vi "Client2.vi"() -> ()   [LabVIEW 2016]
uses:
  <vilib>/Utility/tcp.llb/UDP Multicast Read-Only Open.vi
panel:
  out "MA_Validation":u8
  out "IsNotConnected?":bool
  in  "LeaveServer":bool
  out "Greetings":string
  in  "Exit":bool
  out "MulticastAddress":string
  out "AuthKey":string
  in  "Connect":bool
  in  "Server Port":u32
  in  "Server IP":string
  in  "Send":bool
  in  "Chat_Insert":string
  out "Chat":string
  # "Server IP-Adress"
  # "Server Port"
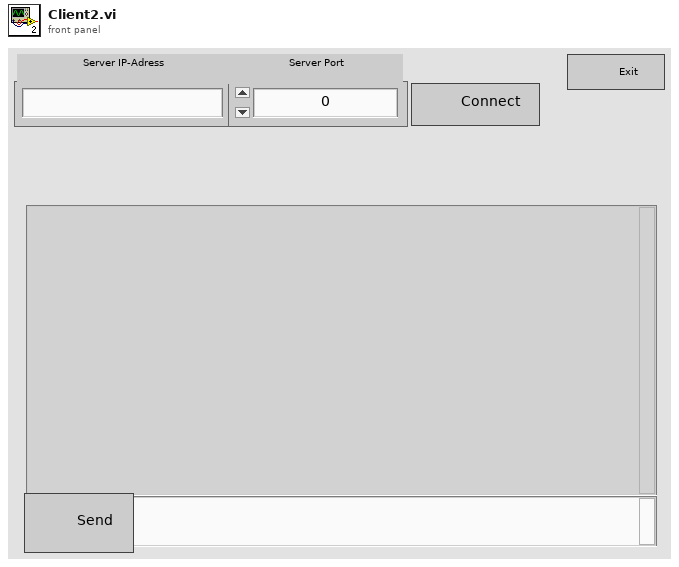
[diagram p1: front panel]
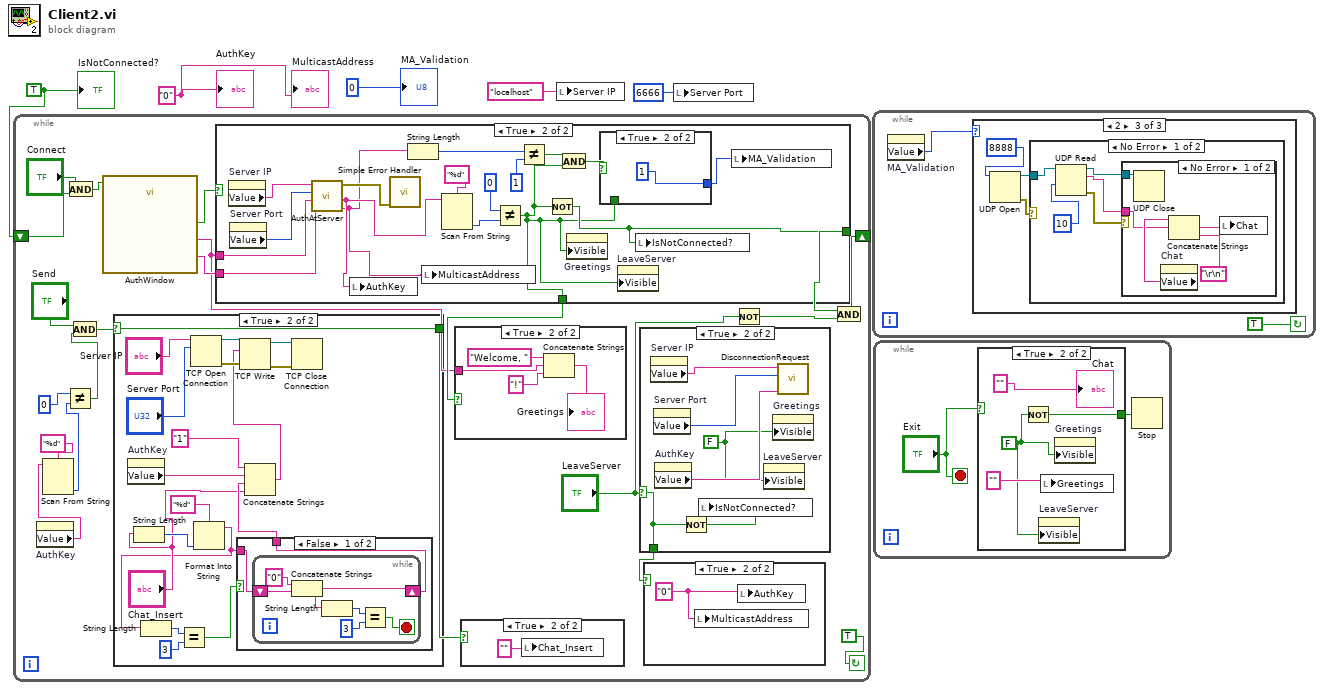
[diagram p0: block diagram]
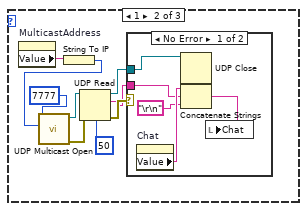
[diagram p3: hidden frame]
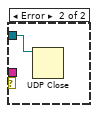
[diagram p5: hidden frame]
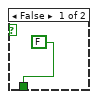
[diagram p9: hidden frame]
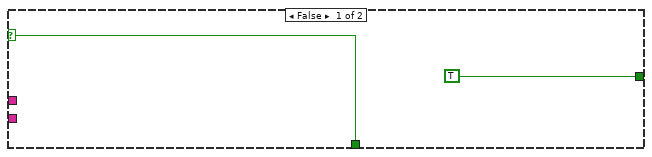
[diagram p14: hidden frame]
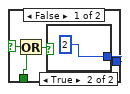
[diagram p15: hidden frame]
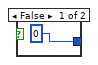
[diagram p16: hidden frame]
diagram:
  w1 = TRUE
  w2 = "0"
  n1 = while {
    shift-right: [w9] -> _
    shift-left: w1 -> [w8]
    stop <- TRUE continue-if-true
    n2 = property on="AuthKey" class="Str"() -> ("Value"=w20:string)  [unwired: 2 in, 2 out]
    n3 = Scan From String(format string="%d", input string=w20) -> (output 1=w18:i32)  [unwired: 3 in, 3 out]
    n4 = Not Equal?(x=0, y=w18) -> (x != y?=w15:bool)
    n5 = And(x="Connect", y=w8) -> (x .and. y?=w13:bool)
    n6 = And(x="Send", y=w15) -> (x .and. y?=w16:bool)
    n7 = call "AuthWindow.vi"("Enable"=w13) -> ("Password"=w23:string, "Login"=w22:string, "Enter"=w21:bool)  [unwired: 15 in, 1 out]
    n8 = case shown="True" w16 {
      selector: w16 -> [w40 w54]
      tunnel: [w40 w54] -> w25
      frame False {
      }
      frame True {
        n9 = property on="AuthKey" class="Str"() -> ("Value"=w45:string)  [unwired: 2 in, 2 out]
        n10 = String Length(string="Chat_Insert") -> (length=w56:i32)
        n11 = TCP Open Connection(address="Server IP", remote port or service name="Server Port") -> (connection ID=w46:refnum<k5>, error out=w47:errorcluster)  [unwired: 3 in]
        n12 = Format Into String(format string="%d", w56) -> (resulting string=w48:string)  [unwired: 2 in, 1 out]
        n13 = String Length(string=w48) -> (length=w52:i32)
        n14 = Equal?(x=w52, y=3) -> (x = y?=w51:bool)
        n15 = case shown="False" w51 {
          tunnel: w48 -> [w60 w67]
          tunnel: [w59 w67] -> w50
          frame False {
            n16 = while {
              shift-right: [w62] -> w59
              shift-left: w60 -> [w66]
              stop <- w61 stop-if-true
              n17 = Concatenate Strings("0", w66) -> (w62:string)
              n18 = String Length(string=w62) -> (length=w63:i32)
              n19 = Equal?(x=w63, y=3) -> (x = y?=w61:bool)
            }
          }
          frame True {
          }
        }
        n20 = Concatenate Strings("1", w45, w50, "Chat_Insert") -> (w43:string)
        n21 = TCP Write(connection ID=w46, data in=w43, error in (no error)=w47) -> (connection ID out=w42:refnum<k5>, error out=w41:errorcluster)  [unwired: 1 in, 1 out]
        n22 = TCP Close Connection(connection ID=w42, error in (no error)=w41) -> ()  [unwired: 1 in, 2 out]
      }
    }
    n23 = case shown="True" w21 {
      selector: w21 -> [w69 _]
      tunnel: w22 -> [_ w83]
      tunnel: w23 -> [_ w82]
      tunnel: [w69 w72] -> w24
      tunnel: [TRUE w77] -> w6
      frame False {
      }
      frame True {
        n24 = property on="Server IP" class="Str"() -> ("Value"=w85:string)  [unwired: 2 in, 2 out]
        n25 = property on="Server Port" class="DigNum (strict)"() -> ("Value"=w84:u32)  [unwired: 2 in, 2 out]
        n26 = call "AuthAtServer.vi"("password"=w82, "login"=w83, "Port"=w84, "Adress"=w85) -> ("MulticastAdress"=w75:string, "AuthKey"=w78:string, "error out"=w86:errorcluster)  [unwired: 5 in]
        n27 = local write "AuthKey"(w78) -> ()
        n28 = call <vilib>:"Simple Error Handler.vi"("error in (no error)"=w86) -> ()  [unwired: 4 in, 5 out]
        n29 = String Length(string=w75) -> (length=w74:i32)
        n30 = local write "MulticastAddress"(w75) -> ()
        n31 = Scan From String(format string="%d", input string=w78) -> (output 1=w80:i32)  [unwired: 3 in, 3 out]
        n32 = Not Equal?(x=0, y=w80) -> (x != y?=w72:bool)
        n33 = Not Equal?(x=w74, y=1) -> (x != y?=w71:bool)
        n34 = Not(x=w72) -> (.not. x?=w77:bool)
        n35 = And(x=w71, y=w72) -> (x .and. y?=w73:bool)
        n36 = property on="Greetings" class="Str"("Visible"=w72) -> ()  [unwired: 2 in, 2 out]
        n37 = case shown="True" w73 {
          selector: w73 -> [w87 _]
          tunnel: [w90 1] -> w70
          tunnel: w72 -> [w89 _]
          frame False {
            n38 = Or(x=w87, y=w89) -> (x .or. y?=w88:bool)
            n39 = case shown="True" w88 {
              tunnel: [0 2] -> w90
              frame False {
              }
              frame True {
              }
            }
          }
          frame True {
          }
        }
        n40 = property on="LeaveServer" class="Bool"("Visible"=w72) -> ()  [unwired: 2 in, 2 out]
        n41 = local write "IsNotConnected?"(w77) -> ()
        n42 = local write "MA_Validation"(w70) -> ()
      }
    }
    n43 = case shown="True" w24 {
      tunnel: w22 -> [_ w37]
      frame False {
      }
      frame True {
        n44 = Concatenate Strings("Welcome, ", w37, "!") -> (→"Greetings":string)
      }
    }
    n45 = case shown="True" w25 {
      frame False {
      }
      frame True {
        n46 = local write "Chat_Insert"("") -> ()
      }
    }
    n47 = case shown="True" "LeaveServer" {
      selector: "LeaveServer" -> [_ w31]
      tunnel: [FALSE w31] -> w11
      frame False {
      }
      frame True {
        w29 = FALSE
        n48 = property on="Server IP" class="Str"() -> ("Value"=w34:string)  [unwired: 2 in, 2 out]
        n49 = property on="Server Port" class="DigNum (strict)"() -> ("Value"=w33:u32)  [unwired: 2 in, 2 out]
        n50 = property on="AuthKey" class="Str"() -> ("Value"=w32:string)  [unwired: 2 in, 2 out]
        n51 = Not(x=w31) -> (.not. x?=w30:bool)
        n52 = local write "IsNotConnected?"(w30) -> ()
        n53 = property on="LeaveServer" class="Bool"("Visible"=w29) -> ()  [unwired: 2 in, 2 out]
        n54 = property on="Greetings" class="Str"("Visible"=w29) -> ()  [unwired: 2 in, 2 out]
        n55 = call "DisconnectionRequest.vi"("AuthKey"=w32, "Server Port"=w33, "Server IP"=w34) -> ()  [unwired: 9 in]
      }
    }
    n56 = case shown="True" w11 {
      frame False {
      }
      frame True {
        w27 = "0"
        n57 = local write "MulticastAddress"(w27) -> ()
        n58 = local write "AuthKey"(w27) -> ()
      }
    }
    n59 = Not(x="LeaveServer") -> (.not. x?=w7:bool)
    n60 = And(x=w6, y=w7) -> (x .and. y?=w9:bool)
  }
  n61 = local write "Server IP"("localhost") -> ()
  n62 = local write "Server Port"(u16 6666) -> ()
  n63 = while {
    stop <- TRUE continue-if-true
    n64 = property on="MA_Validation" class="DigNum (strict)"() -> ("Value"=w94:u8)  [unwired: 2 in, 2 out]
    n65 = case shown="2" w94 {
      frame 0, Default {
      }
      frame 1 {
        n66 = property on="MulticastAddress" class="Str"() -> ("Value"=w103:string)  [unwired: 2 in, 2 out]
        n67 = String To IP(1:w103) -> (0:w102:u32)
        n68 = call-poly <vilib>:"UDP Multicast Open.vi"("multicast addr"=w102, "port"=7777) -> ("error out"=w100:errorcluster, "connection ID"=w101:refnum<k16>)  [unwired: 7 in, 1 out]
        n69 = UDP Read(connection ID=w101, timeout ms (25000)=50, 8:w100) -> (data out=w96:string, error out=w97:errorcluster, 3:w98:refnum<k16>)  [unwired: 1 in, 2 out]
        n70 = case shown="No Error" w97 {
          tunnel: w98 -> [w106 _]
          tunnel: w96 -> [w105 _]
          frame No Error {
            n71 = property on="Chat" class="Str"() -> ("Value"=w109:string)  [unwired: 2 in, 2 out]
            n72 = UDP Close(connection ID=w106) -> ()  [unwired: 1 in, 2 out]
            n73 = Concatenate Strings(w109, w105, "\r\n") -> (w108:string)
            n74 = local write "Chat"(w108) -> ()
          }
          frame Error {
          }
        }
      }
      frame 2 {
        n75 = UDP Open(11:8888) -> (port=w111:refnum<k16>, 0:w112:errorcluster)  [unwired: 4 in, 1 out]
        n76 = case shown="No Error" w112 {
          tunnel: w111 -> [w117 _]
          frame No Error {
            n77 = UDP Read(connection ID=w117, timeout ms (25000)=10) -> (data out=w114:string, error out=w115:errorcluster, 3:w116:refnum<k16>)  [unwired: 2 in, 2 out]
            n78 = case shown="No Error" w115 {
              tunnel: w116 -> [w119 w123]
              tunnel: w114 -> [w118 _]
              frame No Error {
                n79 = UDP Close(connection ID=w119) -> ()  [unwired: 1 in, 2 out]
                n80 = property on="Chat" class="Str"() -> ("Value"=w122:string)  [unwired: 2 in, 2 out]
                n81 = Concatenate Strings(w122, w118, "\r\n") -> (w120:string)
                n82 = local write "Chat"(w120) -> ()
              }
              frame Error {
                n83 = UDP Close(connection ID=w123) -> ()  [unwired: 1 in, 2 out]
              }
            }
          }
          frame Error {
          }
        }
      }
    }
  }
  n84 = while {
    stop <- "Exit" stop-if-true
    n85 = case shown="True" "Exit" {
      selector: "Exit" -> [w126 _]
      tunnel: [w126 w129] -> w124
      frame False {
      }
      frame True {
        w128 = FALSE
        n86 = Not(x=w128) -> (.not. x?=w129:bool)
        n87 = property on="LeaveServer" class="Bool"("Visible"=w128) -> ()  [unwired: 2 in, 2 out]
        n88 = local write "Greetings"("") -> ()
        n89 = property on="Greetings" class="Str"("Visible"=w128) -> ()  [unwired: 2 in, 2 out]
        "Chat" <- ""
      }
    }
    n90 = Stop(stop? (T)=w124) -> ()
  }
  "MulticastAddress" <- w2
  "AuthKey" <- w2
  "IsNotConnected?" <- w1
  "MA_Validation" <- 0
